vi "Create (Child Name).vi"(7 "Ignore Missing (F)":bool, 8 "error in (no error)":errorcluster, 10 "Child Name":string="Config", 11 "Parent":refnum<class "VolatusConfigElement.lvclass">) -> (0 "error out":errorcluster, 3 "VolatusConfigElement out":refnum<class "VolatusConfigElement.lvclass">)   [LabVIEW 2023, in "VolatusConfig.lvlib" / "VolatusConfigElement.lvclass"]
uses:
  VolatusConfigElement.lvclass
  VolatusConfigElement.lvclass/VolatusConfigElement.ctl
  lv-cdm/CDM-Config/Config Element/Config Element.lvclass
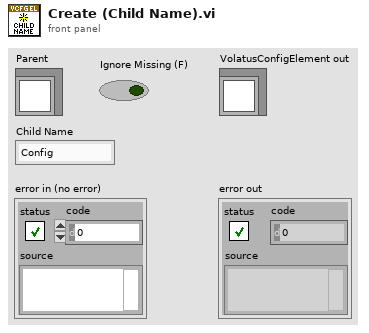
[diagram p1: front panel]
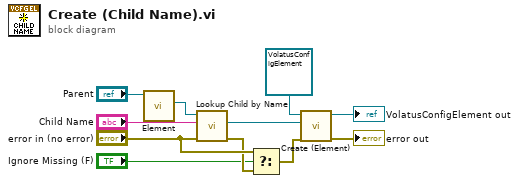
[diagram p0: block diagram]
diagram:
  n1 = call "Element.vi"("VolatusConfigElement in"="Parent") -> ("Element"=w6:refnum<class "Config Element.lvclass">)  [unwired: 9 in, 1 out]
  n2 = call "Lookup Child by Name.vi"("error in (no error)"="error in (no error)", "Name"="Child Name", "Config Element in"=w6) -> ("error out"=w3:errorcluster, "Child"=w10:refnum<class "Config Element.lvclass">)  [unwired: 5 in, 2 out]
  n3 = Select(t="error in (no error)", s="Ignore Missing (F)", f=w3) -> (s? t:f=w1:errorcluster)
  n4 = call "Create (Element).vi"("error in (no error)"=w1, "Element"=w10, "VolatusConfigElement in"=refnum<class "VolatusConfigElement.lvclass"> refnum) -> ("error out"=→"error out":errorcluster, "VolatusConfigElement out"=→"VolatusConfigElement out":refnum<class "VolatusConfigElement.lvclass">)  [unwired: 7 in]
